vi "Read out INTERLOCK Mode.vi"(8 "error in (no error)":errorcluster, 11 "BoardHandle":T1) -> (0 "error out":errorcluster, 2 "Interlock Mode":string, 3 "BoardHandle out":T1)   [LabVIEW 2019, in "CAEN PSM.lvlib"]
doc: "This function returns interlock mode"
uses:
  Users/pcmmegas02/Downloads/CAEN_PSM-InstrumentDriver-1.0.2/CAEN PSM/CAEN PSM.lvlib
  Users/pcmmegas02/Downloads/CAEN_PSM-InstrumentDriver-1.0.2/CAEN PSM/Private/BoardHandle.ctl
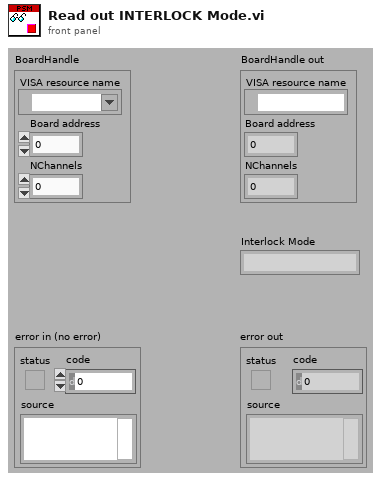
[diagram p1: front panel]
types:
  T1 = typedef "CAEN PSM.lvlib/BoardHandle.ctl" = cluster{"VISA resource name":refnum<visa-resource-name>, "Board address":u8, "NChannels":u8}
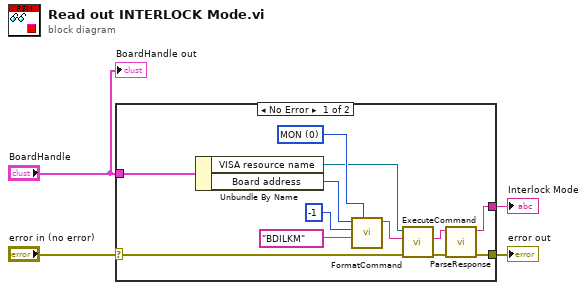
[diagram p0: block diagram]
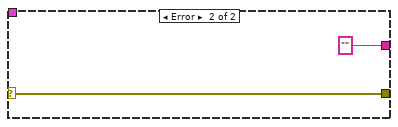
[diagram p2: hidden frame]
diagram:
  n1 = case shown="No Error" "error in (no error)" {
    selector: "error in (no error)" -> [w8 w18]
    tunnel: [w11 w18] -> w3
    tunnel: "BoardHandle" -> [w9 _]
    tunnel: [w5 "" ("val")] -> w1
    frame No Error {
      w15 = u8 0 items=["MON", "SET"] ("CMD")
      n2 = Unbundle By Name(w9) -> ("VISA resource name"=w14:refnum<visa-resource-name>, "Board address"=w16:u8)
      n3 = call "FormatCommand.vi"("CMD (MON)"=w15, "PAR"="BDILKM", "CH"=i8 -1, "BD (0)"=w16) -> ("cmd"=w13:string)  [unwired: 7 in]
      n4 = call "ExecuteCommand.vi"("error in (no error)"=w8, "Command"=w13, "VISA resource name"=w14) -> ("error out"=w12:errorcluster, "Response"=w10:string)  [unwired: 6 in, 1 out]
      n5 = call "ParseResponse.vi"("error in (no error)"=w12, "Response"=w10) -> ("error out"=w11:errorcluster, "val"=w5:string)  [unwired: 6 in, 2 out]
    }
    frame Error {
    }
  }
  "error out" <- w3
  "Interlock Mode" <- w1
  "BoardHandle out" <- "BoardHandle"
